vi "Send onStatusUpdated.vi"(7 "Message Priority (Normal)":T2=enum."Normal", 8 "error in (no error)":errorcluster, 10 "StatusRecord":T1, 11 "Message Enqueuer":refnum<class "Message Enqueuer.lvclass">) -> (0 "error out":errorcluster, 3 "Message Enqueuer out":refnum<class "Message Enqueuer.lvclass">)   [LabVIEW 2020, in "CameraTestingUI.lvlib" / "onStatusUpdated Msg.lvclass"]
doc: "This VI sends the message to an actor."
uses:
  onStatusUpdated Msg.lvclass
  <vilib>/ActorFramework/Message Enqueuer/Message Enqueuer.lvclass
  <vilib>/ActorFramework/Message Enqueuer/Message Priority.ctl
  ICameraTesting/TypeDef/StatusRecord.ctl
  C:/Program Files (x86)/National Instruments/LabVIEW 2020/vi.lib/ActorFramework/Message/Message.lvclass
  onStatusUpdated Msg.lvclass/onStatusUpdated Msg.ctl
  <vilib>/ActorFramework/Message Enqueuer/Message Enqueuer.lvclass/Message Enqueuer.ctl
  <vilib>/ActorFramework/Message Priority Queue/Priority Enqueue.vi
  ICameraTesting/TypeDef/ICameraTesting_typedef.lvlib
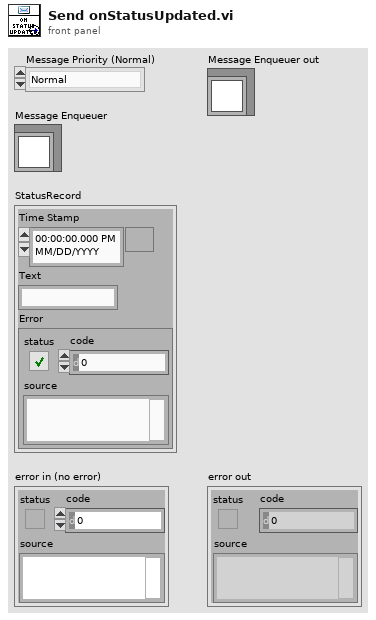
[diagram p1: front panel]
types:
  T1 = typedef "ICameraTesting_typedef.lvlib/StatusRecord.ctl" = cluster{"Time Stamp":timestamp, "Text":string, "Error":errorcluster}
  T2 = typedef "Actor Framework.lvlib/Message Enqueuer.lvclass/Message Priority.ctl" = enum16{"Low", "Normal", "High"}
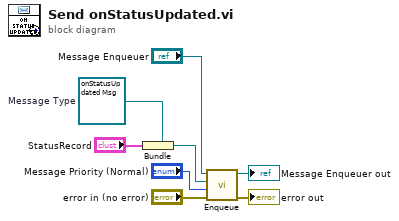
[diagram p0: block diagram]
diagram:
  w5 = refnum<class "onStatusUpdated Msg.lvclass"> refnum  # Message Type
  n1 = Bundle(cluster=w5, "StatusRecord") -> (w4:refnum<class "onStatusUpdated Msg.lvclass">)
  n2 = call <vilib>:"Enqueue.vi"("error in (no error)"="error in (no error)", "Message Priority (Normal)"="Message Priority (Normal)", "Message"=w4, "Message Enqueuer in"="Message Enqueuer") -> ("error out"=→"error out":errorcluster, "Message Enqueuer out"=→"Message Enqueuer out":refnum<class "Message Enqueuer.lvclass">)  [unwired: 6 in]
